vi "Program path (SubVI).vi"() -> (3 "Trap clusters":T1[](array[typedef]))   [LabVIEW 2011]
uses:
  Trap cluster.ctl
panel:
  out "trap cluster":T1
  in  "N traps":i32
  in  "stop":bool
  in  "Z position":dbl
  in  "I stop":dbl[](array[numeric])
  in  "I start":dbl[](array[numeric])
  in  "Y stop":dbl[](array[numeric])
  in  "Y start":dbl[](array[numeric])
  in  "X stop":dbl[](array[numeric])
  in  "X start":dbl[](array[numeric])
  in  "dI":dbl
  in  "dX and dY":dbl
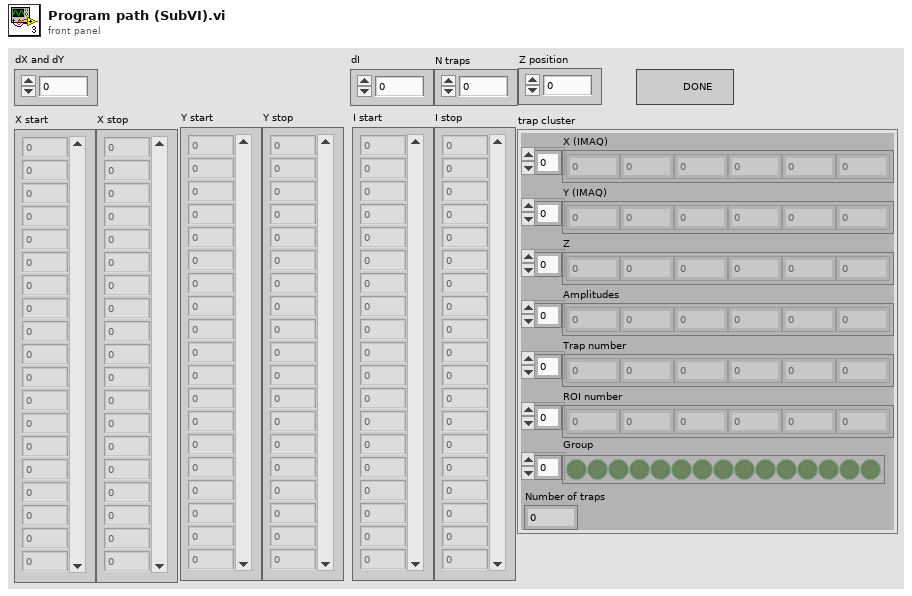
[diagram p1: front panel]
types:
  T1 = typedef "Trap cluster.ctl" = cluster{"X (IMAQ)":dbl[], "Y (IMAQ)":dbl[], "Z":dbl[], "Amplitudes":dbl[], "Trap number":i32[], "ROI number":i32[], "Number of traps":i32, "Group":bool[]}
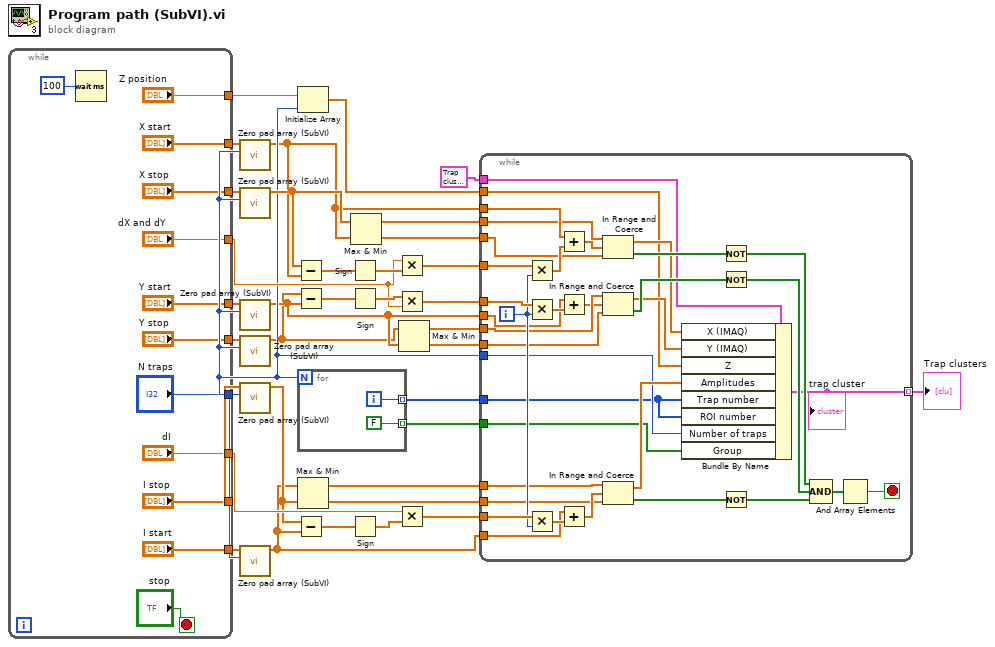
[diagram p0: block diagram]
diagram:
  n1 = while {
    tunnel: ["dX and dY"] -> w29
    tunnel: ["dI"] -> w27
    tunnel: ["X stop"] -> w12
    tunnel: ["X start"] -> w10
    tunnel: ["Y stop"] -> w5
    tunnel: ["Y start"] -> w8
    tunnel: ["I stop"] -> w4
    tunnel: ["Z position"] -> w19
    tunnel: ["I start"] -> w2
    tunnel: ["N traps"] -> w11
    stop <- "stop" stop-if-true
    n2 = Wait (ms)(milliseconds to wait=u32 100) -> ()  [unwired: 1 out]
  }
  n3 = call "Zero pad array (SubVI).vi"("length"=w11, "Array in"=w10) -> ("Array out"=w9:dbl[])  [unwired: 9 in]
  n4 = call "Zero pad array (SubVI).vi"("length"=w11, "Array in"=w12) -> ("Array out"=w13:dbl[])  [unwired: 9 in]
  n5 = call "Zero pad array (SubVI).vi"("length"=w11, "Array in"=w8) -> ("Array out"=w7:dbl[])  [unwired: 9 in]
  n6 = call "Zero pad array (SubVI).vi"("length"=w11, "Array in"=w5) -> ("Array out"=w6:dbl[])  [unwired: 9 in]
  n7 = call "Zero pad array (SubVI).vi"("length"=w11, "Array in"=w4) -> ("Array out"=w3:dbl[])  [unwired: 9 in]
  n8 = call "Zero pad array (SubVI).vi"("length"=w11, "Array in"=w2) -> ("Array out"=w1:dbl[])  [unwired: 9 in]
  n9 = Subtract(x=w13, y=w9) -> (x-y=w31:dbl[])
  n10 = Subtract(x=w6, y=w7) -> (x-y=w30:dbl[])
  n11 = Subtract(x=w3, y=w1) -> (x-y=w28:dbl[])
  n12 = Initialize Array(w19, w11) -> (w18:dbl[])
  n13 = for {
    N: w11 -> [_]
    tunnel: [w50] -> w17 mode=indexing
    tunnel: [FALSE ("Boolean")] -> w16 mode=indexing
    i -> [w50]
  }
  n14 = Max & Min(x=w1, y=w3) -> (max(x,y)=w22:dbl[], min(x,y)=w21:dbl[])
  n15 = Sign(1:w31) -> (0:w36:dbl[])
  n16 = Sign(1:w30) -> (0:w35:dbl[])
  n17 = Sign(1:w28) -> (0:w32:dbl[])
  n18 = Max & Min(x=w13, y=w9) -> (max(x,y)=w26:dbl[], min(x,y)=w25:dbl[])
  n19 = Multiply(x=w29, y=w36) -> (x*y=w34:dbl[])
  n20 = Multiply(x=w35, y=w29) -> (x*y=w33:dbl[])
  n21 = Multiply(x=w27, y=w32) -> (x*y=w14:dbl[])
  n22 = Max & Min(x=w6, y=w7) -> (max(x,y)=w24:dbl[], min(x,y)=w23:dbl[])
  n23 = while {
    tunnel: w34 -> [w86]
    tunnel: w33 -> [w85]
    tunnel: w14 -> [w84]
    tunnel: w9 -> [w80]
    tunnel: w7 -> [w79]
    tunnel: w1 -> [w78]
    tunnel: w26 -> [w76]
    tunnel: w25 -> [w75]
    tunnel: w24 -> [w74]
    tunnel: w23 -> [w73]
    tunnel: w22 -> [w69]
    tunnel: w21 -> [w68]
    tunnel: T1 {"X (IMAQ)"=[], "Y (IMAQ)"=[], "Z"=[], "Amplitudes"=[], "Trap number"=[], "ROI number"=[], "Number of traps"=0, "Group"=[]} ("output cluster 3") -> [w59]
    tunnel: [w58] -> w15 mode=indexing
    tunnel: w18 -> [w54]
    tunnel: w17 -> [w52]
    tunnel: w11 -> [w53]
    tunnel: w16 -> [w51]
    i -> [w83]
    stop <- w63 stop-if-true
    n24 = Multiply(x=w86, y=w83) -> (x*y=w77:dbl[])
    n25 = Multiply(x=w85, y=w83) -> (x*y=w81:dbl[])
    n26 = Multiply(x=w84, y=w83) -> (x*y=w82:dbl[])
    n27 = Add(x=w80, y=w77) -> (x+y=w71:dbl[])
    n28 = Add(x=w79, y=w81) -> (x+y=w72:dbl[])
    n29 = Add(x=w78, y=w82) -> (x+y=w70:dbl[])
    n30 = In Range and Coerce(upper limit=w76, x=w71, lower limit=w75) -> (coerced(x)=w57:dbl[], In Range?=w67:bool[])
    n31 = In Range and Coerce(upper limit=w74, x=w72, lower limit=w73) -> (coerced(x)=w56:dbl[], In Range?=w66:bool[])
    n32 = In Range and Coerce(upper limit=w69, x=w70, lower limit=w68) -> (coerced(x)=w55:dbl[], In Range?=w65:bool[])
    n33 = Bundle By Name(cluster=w59, "X (IMAQ)"=w57, "Y (IMAQ)"=w56, "Z"=w54, "Amplitudes"=w55, "Trap number"=w52, "ROI number"=w52, "Number of traps"=w53, "Group"=w51) -> (w58:T1)
    "trap cluster" <- w58
    n34 = Not(x=w67) -> (.not. x?=w62:bool[])
    n35 = Not(x=w66) -> (.not. x?=w61:bool[])
    n36 = Not(x=w65) -> (.not. x?=w60:bool[])
    n37 = Compound Arithmetic op=AND(w62, w61, w60) -> (w64:bool[])
    n38 = And Array Elements(Boolean array=w64) -> (logical AND=w63:bool)
  }
  "Trap clusters" <- w15
